vi "Fausse couleur.vi"() -> ()   [LabVIEW 2026]
uses:
  <vilib>/Analysis/1siggen.llb/Ramp Pattern by Samples.vi
  <vilib>/Analysis/NI_AALBase.lvlib
panel:
  out "taille(s)":i32
  out "Ramp Pattern":dbl[](array[numeric]) caption="Motif de rampe"
  out "Tableau 2":u8[](array[numeric])
  out "Tableau":u32[](array[colorbox])
  out "b":dbl
  out "g":dbl
  out "r":dbl
  out "t":dbl
  out "B":u8
  out "G":u8
  out "R":u8
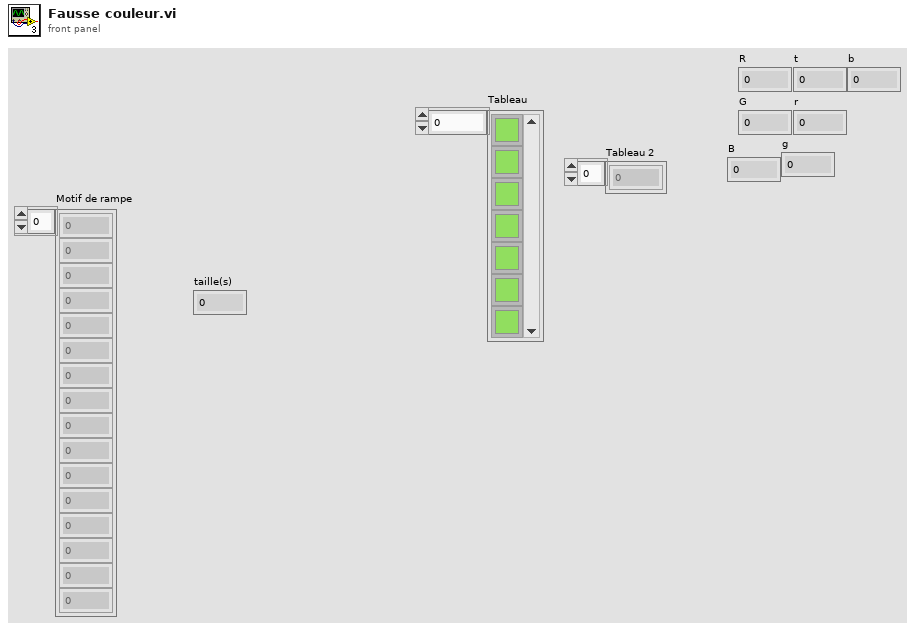
[diagram p1: front panel]
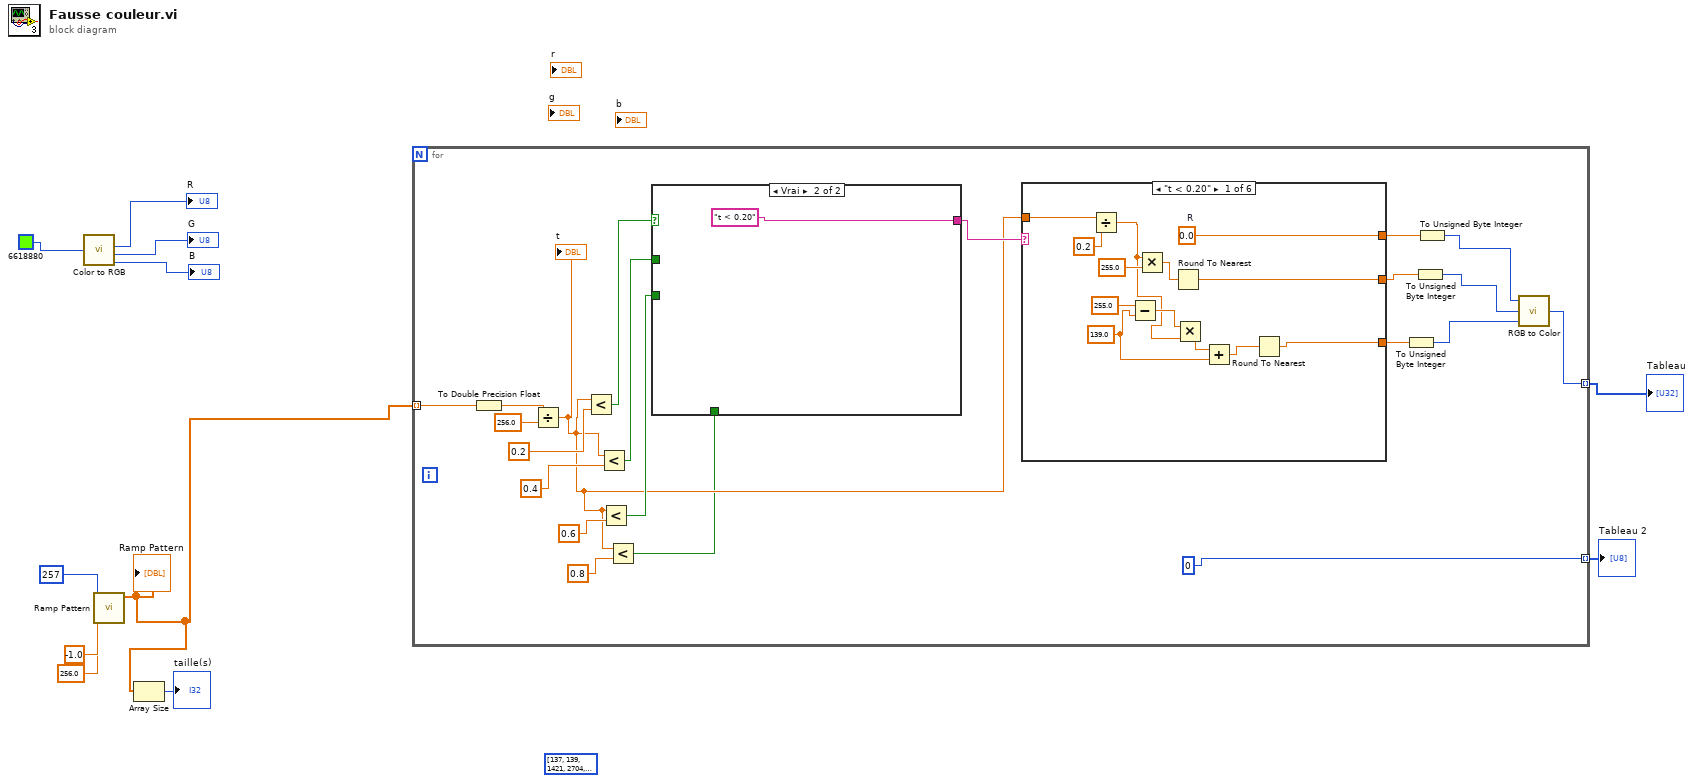
[diagram p0: block diagram]
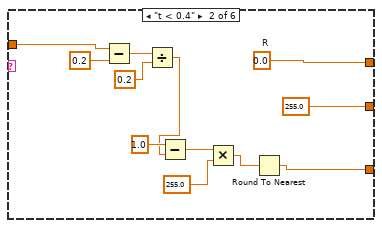
[diagram p2: hidden frame]
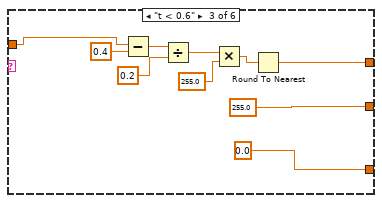
[diagram p3: hidden frame]
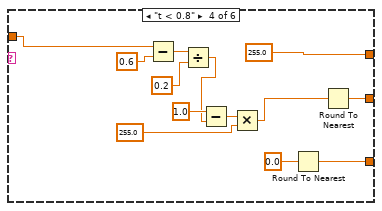
[diagram p4: hidden frame]
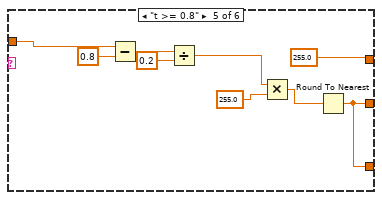
[diagram p5: hidden frame]
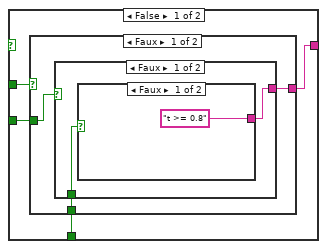
[diagram p7: hidden frame]
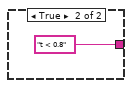
[diagram p8: hidden frame]
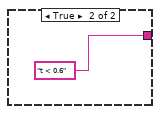
[diagram p9: hidden frame]
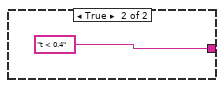
[diagram p10: hidden frame]
diagram:
  (unwired) u32[] [137, 139, 1421, 2704, 3986, 5268, 6550, 7833, 9115, 10397, 11679, 12962, 14244, 15526, 16809, 18091, 19373, 20655, 21938, 23220, 24502, 25784, 27067, 28349, 29631, 30914, 32196, 33478, 34760, 36043, 37325, 38607, 39890, 41172, 42454, 43736, 45019, 46301, 47583, 48865, 50148, 51430, 52712, 53995, 55277, 56559, 57841, 59124, 60406, 61688, 62970, 64253, 65535, 65530, 65525, 65520, 65515, 65510, 65505, 65500, 65495, 65490, 65485, 65480, 65475, 65470, 65465, 65460, 65455, 65450, 65445, 65440, 65435, 65430, 65425, 65420, 65415, 65410, 65405, 65400, 65395, 65390, 65385, 65380, 65375, 65370, 65365, 65360, 65355, 65350, 65345, 65340, 65335, 65330, 65325, 65320, 65315, 65310, 65305, 65300, 65295, 65290, 65285, 65280, 392960, 720640, 1048320, 1376000, 1703680, 2031360, 2359040, 2686720, 3014400, 3342080, 3669760, 3997440, 4325120, 4652800, 4980480, 5308160, 5635840, 5963520, 6291200, 6618880, 6946560, 7274240, 7601920, 7929600, 8257280, 8584960, 8912640, 9240320, 9568000, 9895680, 10223360, 10551040, 10878720, 11206400, 11534080, 11861760, 12189440, 12517120, 12844800, 13172480, 13500160, 13827840, 14155520, 14483200, 14810880, 15138560, 15466240, 15793920, 16121600, 16449280, 16776960, 16775680, 16774400, 16773120, 16771840, 16770560, 16769280, 16768000, 16766720, 16765440, 16764160, 16762880, 16761600, 16760320, 16759040, 16757760, 16756480, 16755200, 16753920, 16752640, 16751360, 16750080, 16748800, 16747520, 16746240, 16744960, 16743680, 16742400, 16741120, 16739840, 16738560, 16737280, 16736000, 16734720, 16733440, 16732160, 16730880, 16729600, 16728320, 16727040, 16725760, 16724480, 16723200, 16721920, 16720640, 16719360, 16718080, 16716800, 16715520, 16714240, 16712960, 16711680, 16712965, 16714250, 16715535, 16716820, 16718105, 16719390, 16720675, 16721960, 16723245, 16724530, 16725815, 16727100, 16728385, 16729670, 16730955, 16732240, 16733525, 16734810, 16736095, 16737380, 16738665, 16739950, 16741235, 16742520, 16743805, 16745090, 16746375, 16747660, 16748945, 16750230, 16751515, 16752800, 16754085, 16755370, 16756655, 16757940, 16759225, 16760510, 16761795, 16763080, 16764365, 16765650, 16766935, 16768220, 16769505, 16770790, 16772075, 16773360, 16774645, 16775930, 16777215] ("Tableau 3")
  n1 = call <vilib>:"Color to RGB.vi"("Color"=u32 6618880 ("color(black)")) -> ("R"=→"R":u8, "G"=→"G":u8, "B"=→"B":u8)  [unwired: 1 out]
  n2 = call-poly <vilib>:"Ramp Pattern.vi"("start"=-1.0, "end"=256.0, "samples"=257) -> ("Ramp Pattern"=w1:dbl[])  [unwired: 7 in, 1 out]
  "Ramp Pattern" <- w1
  n3 = Array Size(array=w1) -> (size(s)=→"taille(s)":i32)
  n4 = for {
    tunnel: [w17] -> w7 mode=indexing
    tunnel: [u8 0] -> w6 mode=indexing
    tunnel: w1 -> [w12] mode=indexing
    n5 = To Double Precision Float(number=w12) -> (double precision float=w31:dbl)
    n6 = Divide(x=w31, y=256.0) -> (x/y=w15:dbl)
    "t" <- w15
    n7 = Less?(x=w15, y=0.2) -> (x < y?=w29:bool)
    n8 = Less?(x=w15, y=0.4) -> (x < y?=w26:bool)
    n9 = Less?(x=w15, y=0.6) -> (x < y?=w24:bool)
    n10 = Less?(x=w15, y=0.8) -> (x < y?=w14:bool)
    n11 = case shown="Vrai" w29 {
      tunnel: [w93 "t < 0.20"] -> w28
      tunnel: w26 -> [w92 _]
      tunnel: w24 -> [w91 _]
      tunnel: w14 -> [w90 _]
      frame False {
        n12 = case shown="Faux" w92 {
          tunnel: [w96 "t < 0.4"] -> w93
          tunnel: w91 -> [w95 _]
          tunnel: w90 -> [w94 _]
          frame False {
            n13 = case shown="Faux" w95 {
              tunnel: [w98 "t < 0.6"] -> w96
              tunnel: w94 -> [w97 _]
              frame False {
                n14 = case shown="Faux" w97 {
                  tunnel: ["t >= 0.8" "t < 0.8"] -> w98
                  frame False {
                  }
                  frame True {
                  }
                }
              }
              frame True {
              }
            }
          }
          frame True {
          }
        }
      }
      frame True {
      }
    }
    n15 = case shown="\"t < 0.20\"" w28 {
      tunnel: w15 -> [w44 w56 w66 w79 w89 _]
      tunnel: [w43 w53 w60 255.0 ("y") 255.0 ("y") _] -> w23
      tunnel: [w40 255.0 ("y") 255.0 ("y") w71 w81 _] -> w22
      tunnel: [w33 w47 0.0 ("y") w70 w81 _] -> w21
      frame "t < 0.20" {
        w35 = 139.0 ("y")
        w43 = 0.0  # R
        n16 = Divide(x=w44, y=0.2) -> (x/y=w37:dbl)
        n17 = Subtract(x=255.0, y=w35) -> (x-y=w38:dbl)
        n18 = Multiply(x=w37, y=255.0) -> (x*y=w41:dbl)
        n19 = Round To Nearest(number=w41) -> (nearest integer value=w40:dbl)
        n20 = Multiply(x=w38, y=w37) -> (x*y=w36:dbl)
        n21 = Add(x=w36, y=w35) -> (x+y=w34:dbl)
        n22 = Round To Nearest(number=w34) -> (nearest integer value=w33:dbl)
      }
      frame "t < 0.4" {
        w53 = 0.0  # R
        n23 = Subtract(x=w56, y=0.2) -> (x-y=w55:dbl)
        n24 = Divide(x=w55, y=0.2) -> (x/y=w51:dbl)
        n25 = Subtract(x=1.0, y=w51) -> (x-y=w50:dbl)
        n26 = Multiply(x=w50, y=255.0) -> (x*y=w48:dbl)
        n27 = Round To Nearest(number=w48) -> (nearest integer value=w47:dbl)
      }
      frame "t < 0.6" {
        n28 = Subtract(x=w66, y=0.4) -> (x-y=w65:dbl)
        n29 = Divide(x=w65, y=0.2) -> (x/y=w62:dbl)
        n30 = Multiply(x=w62, y=255.0) -> (x*y=w61:dbl)
        n31 = Round To Nearest(number=w61) -> (nearest integer value=w60:dbl)
      }
      frame "t < 0.8" {
        n32 = Subtract(x=w79, y=0.6) -> (x-y=w78:dbl)
        n33 = Divide(x=w78, y=0.2) -> (x/y=w72:dbl)
        n34 = Subtract(x=1.0, y=w72) -> (x-y=w74:dbl)
        n35 = Multiply(x=w74, y=255.0) -> (x*y=w69:dbl)
        n36 = Round To Nearest(number=0.0 ("nombre")) -> (nearest integer value=w70:dbl)
        n37 = Round To Nearest(number=w69) -> (nearest integer value=w71:dbl)
      }
      frame "t >= 0.8" {
        n38 = Subtract(x=w89, y=0.8) -> (x-y=w87:dbl)
        n39 = Divide(x=w87, y=0.2) -> (x/y=w84:dbl)
        n40 = Multiply(x=w84, y=255.0) -> (x*y=w82:dbl)
        n41 = Round To Nearest(number=w82) -> (nearest integer value=w81:dbl)
      }
      frame Default {
      }
    }
    n42 = To Unsigned Byte Integer(number=w21) -> (unsigned 8bit integer=w18:u8)
    n43 = To Unsigned Byte Integer(number=w22) -> (unsigned 8bit integer=w19:u8)
    n44 = To Unsigned Byte Integer(number=w23) -> (unsigned 8bit integer=w20:u8)
    n45 = call <vilib>:"RGB to Color.vi"("B"=w18, "G"=w19, "R"=w20) -> ("Color"=w17:u32)
  }
  "Tableau" <- w7
  "Tableau 2" <- w6
